vi "Write RectName Ref.vi"(8 "error in (no error)":errorcluster, 10 "RectName Ref":refnum<vi>, 11 "UEF Handler2 in":refnum<class "UEF Handler2.lvclass">) -> (0 "error out":errorcluster, 3 "UEF Handler2 out":refnum<class "UEF Handler2.lvclass">)   [LabVIEW 2015, in "UEF Handler2.lvclass"]
uses:
  UEF Handler2.lvclass
  UEF Handler2.lvclass/UEF Handler2.ctl
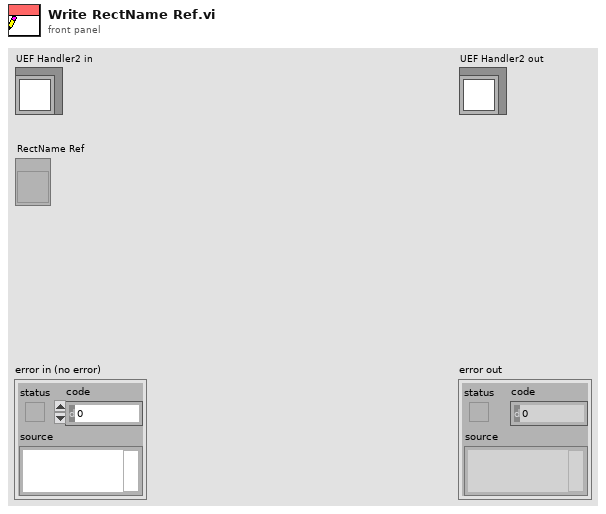
[diagram p1: front panel]
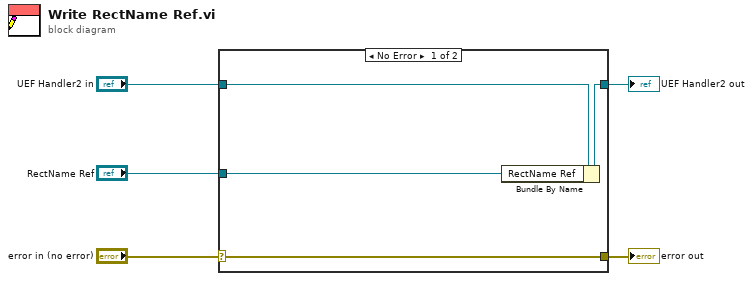
[diagram p0: block diagram]
diagram:
  n1 = case shown="No Error" "error in (no error)" {
    selector: "error in (no error)" -> [w9 w10]
    tunnel: [w9 w10] -> w4
    tunnel: [w7 w11] -> w2
    tunnel: "UEF Handler2 in" -> [w8 w11]
    tunnel: "RectName Ref" -> [w6 _]
    frame No Error {
      n2 = Bundle By Name(cluster=w8, "RectName Ref"=w6) -> (w7:refnum<class "UEF Handler2.lvclass">)
    }
    frame Error {
    }
  }
  "error out" <- w4
  "UEF Handler2 out" <- w2
